vi "CheckQT.vi"() -> (1 "success?":bool)   [LabVIEW 2012]
uses:
  <userlib>/ImageProcessing/QTLIB_2595_LV86/QT_Info.ctl
  <userlib>/ImageProcessing/QTLIB_2595_LV86/QT_Digitizer.ctl
  <userlib>/ImageProcessing/QTLIB_2595_LV86/QT_Private.ctl
panel:
  out "QT Version":string
  out "QT Info":T1={"CIN info"="© Chris 94-2002, QT Fat-CIN, rev: 2549, FATQTCin.c, Oct 24 2002, 14:11:49", "CIN rev ID"=2549.0, "QT Version"="QuickTime v. 502 ", "QT option"=0, "Digitizers\n"=[], "Codec"=["Animation 'rle '", "BMP 'WRLE'", "Cinepak 'cvid'", "Component Video 'yuv2'", "DV - NTSC 'dvc '", "DV - PAL 'dvcp'", "Graphics 'smc '", "H.261 'h261'", "H.263 'h263'", "Motion JPEG A 'mjpa'", "Motion JPEG B 'mjpb'", "None 'raw '", "Photo - JPEG 'jpeg'", "Planar RGB '8BPS'", "PNG 'png '", "Sorenson Video 'SVQ1'", "Sorenson Video 3 'SVQ3'", "TGA 'tga '", "TIFF 'tiff'", "Video 'rpza'"], "reserved 1"=0, "reserved 2"=0} {"Digitizers"."In Flags" format="%.0b"; "Digitizers"."Out Flags" format="%.0b"; "Digitizers"."Inputs" items=["Composite", "S-Video", "RGB", "RGB Synch", "YUV", "YUV Synch", "TV Tuner", "sdiln"]; "CIN rev ID" format="%.2f"}
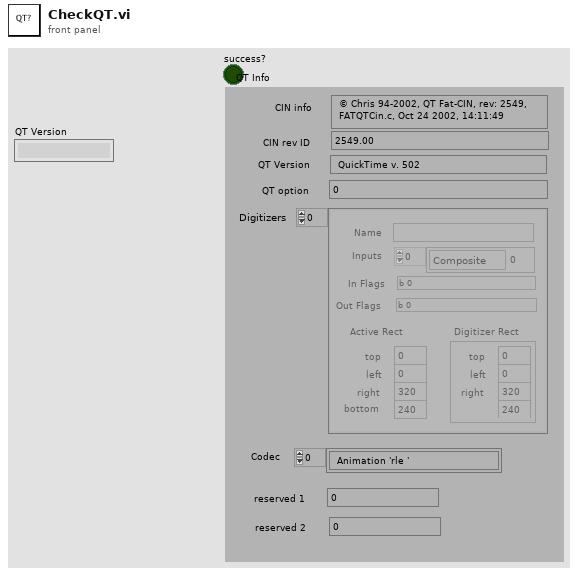
[diagram p1: front panel]
types:
  T1 = typedef "QT_Info.ctl" = cluster{"CIN info":string, "CIN rev ID":dbl, "QT Version":string, "QT option":i32, "Digitizers\n":T2[], "Codec":string[], "reserved 1":i32, "reserved 2":i32}
  T2 = typedef "QT_Digitizer.ctl" = cluster{"Name":string, "Inputs":i32[], "In Flags":i32, "Out Flags":i32, "Digitizer Rect":cluster{"top":i32, "left":i32, "right":i32, "bottom":i32}, "Active Rect":cluster{"top":i32, "left":i32, "right":i32, "bottom":i32}}
  T3 = typedef "QT_Private.ctl" = cluster{"reserved 1":i32, "reserved 2":i32, "reserved 3":i32, "reserved 4":i32}
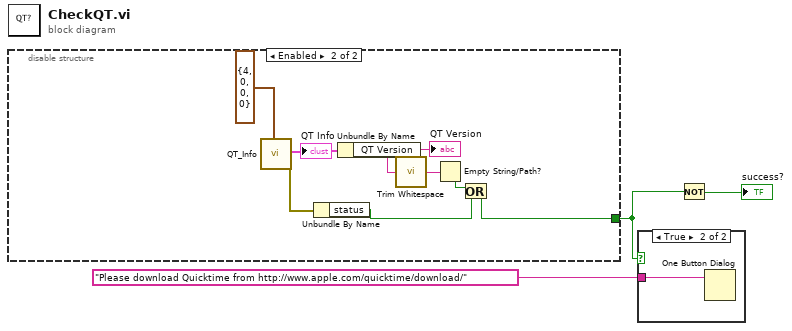
[diagram p0: block diagram]
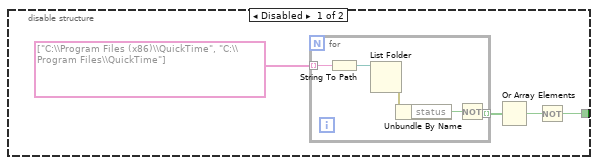
[diagram p2: hidden frame]
diagram:
  n1 = disable-structure shown="Enabled" {
    disable-tunnel: [w4 w13] -> w1
    frame Disabled {
      n2 = for {
        tunnel: string[] ["C:\\Program Files (x86)\\QuickTime", "C:\\Program Files\\QuickTime"] -> [w11] mode=indexing
        tunnel: [w8] -> w6 mode=indexing
        n3 = String To Path(string=w11) -> (path=w12:path)
        n4 = List Folder(path=w12) -> (error out=w9:errorcluster)  [unwired: 3 in, 3 out]
        n5 = Unbundle By Name(w9) -> ("status"=w10:bool)
        n6 = Not(x=w10) -> (.not. x?=w8:bool)
      }
      n7 = Or Array Elements(Boolean array=w6) -> (logical OR=w5:bool)
      n8 = Not(x=w5) -> (.not. x?=w4:bool)
    }
    frame Enabled {
      n9 = call <userlib>:"QT_Info.vi"("Private"=T3 {"reserved 1"=4, "reserved 2"=0, "reserved 3"=0, "reserved 4"=0}) -> ("QT Info"=w18:T1, "error out"=w20:errorcluster)  [unwired: 12 in, 5 out]
      "QT Info" <- w18
      n10 = Unbundle By Name(w20) -> ("status"=w14:bool)
      n11 = Unbundle By Name(w18) -> ("QT Version"=w17:string)
      "QT Version" <- w17
      n12 = call <vilib>:"Trim Whitespace.vi"("string"=w17) -> ("trimmed string"=w16:string)  [unwired: 1 in]
      n13 = Empty String/Path?(string/path=w16) -> (empty?=w15:bool)
      n14 = Or(x=w15, y=w14) -> (x .or. y?=w13:bool)
    }
  }
  n15 = case shown="True" w1 {
    tunnel: "Please download Quicktime from http://www.apple.com/quicktime/download/" ("message") -> [_ w21]
    frame False {
    }
    frame True {
      n16 = One Button Dialog(message=w21) -> ()  [unwired: 1 in, 1 out]
    }
  }
  n17 = Not(x=w1) -> (.not. x?=→"success?":bool)
